vi "SRV_Sensor PARSE_##$A.vi"(0 "Return Data":string) -> (3 "Constant Command":string, 10 "Value":u16)   [LabVIEW 2009]
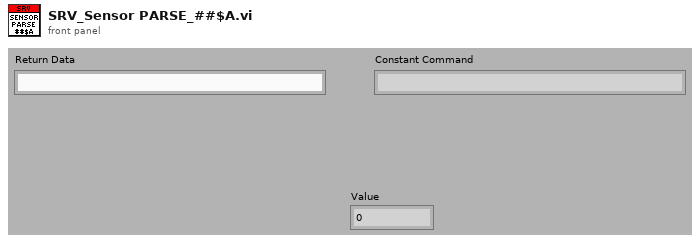
[diagram p1: front panel]
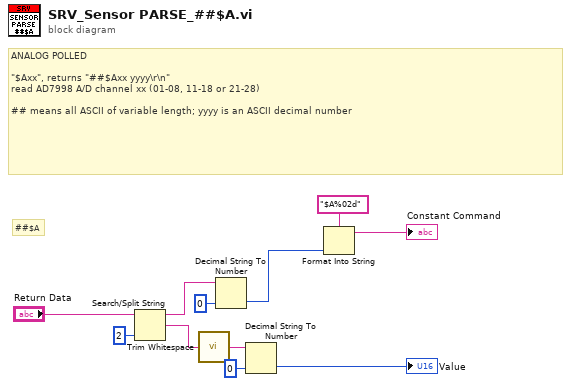
[diagram p0: block diagram]
diagram:
  # "##$A"
  # "ANALOG POLLED\n\n\"$Axx\", returns \"##$Axx yyyy\\r\\n\"\nread AD7998 A/D channel xx (01-08, 11-18 or 21-28)\n\n## means all ASCII of variable length; yyyy is an ASCII decimal number"
  n1 = Search/Split String(string="Return Data", offset (0)=2) -> (substring before match=w9:string, match + rest of string=w7:string)  [unwired: 1 in, 1 out]
  n2 = call <vilib>:"Trim Whitespace.vi"("string"=w7) -> ("trimmed string"=w6:string)  [unwired: 1 in]
  n3 = Decimal String To Number(string=w9, default (0L)=u8 0 ("default (0 I32)")) -> (number=w2:u8)  [unwired: 1 in, 1 out]
  n4 = Decimal String To Number(string=w6, default (0L)=u16 0 ("default (0 I32)")) -> (number=→"Value":u16)  [unwired: 1 in, 1 out]
  n5 = Format Into String(format string="$A%02d", w2) -> (resulting string=→"Constant Command":string)  [unwired: 2 in, 1 out]
